vi "KE622x -- Read Trace Buffer.vi"(0 "Resource In":refnum<visa-resource-name>, 1 "Check For SCPI Errors? (T)":bool=TRUE, 7 "Meas Elements To Return":T1={"Timstamp?"=TRUE, "Reading Num?"=TRUE, "Source Value?"=FALSE, "Compliance?"=FALSE, "Average Voltage?"=FALSE}, 11 "error in (no error)":errorcluster) -> (4 "Resource Out (dupl)":refnum<visa-resource-name>, 8 "Trace Buf":T2 {"Average Voltage (V)" format="%.3p"; "Source Val (A)" format="%.3p"; "Timestamp (secs)" format="%.3f"; "Reading" format="%.3p"}, 15 "error out":errorcluster)   [LabVIEW 2019, in "Keithley 622x.lvlib"]
doc: "Used to read the contents of the trace buffer. The user can select which elements should be returned. Note that the data format of the returned results (ASCII, Single Precision, or Double Precision) is automatically detected and handled appropriately so that the user doesn't need to know this information beforehand."
uses:
  Keithley 622x.lvlib
  Configure/Trace Buf/Low Level/Typedefs/KE622x -- Trace Buf.ctl
  Configure/Format/Typedefs/KE622x -- Optional Meas Elements.ctl
  Configure/Trace Buf/Low Level/Typedefs/KE622x -- Trace Buf Readings Type.ctl
panel:
  out "Select Code Dec":u32 format="%0d"
  out "Max Num Bytes To Read":u32
  out "Read String Length":i32
  out "Select Code Bin":u32 format="%06b"
  out "read buffer":string
  # "*** NOTE:  \"Average Voltage\"\nis only available for Differential\nConductance measurements."
  # "*** NOTE:  \"Average Voltage\"\nis only available for Differential\nConductance measurements."
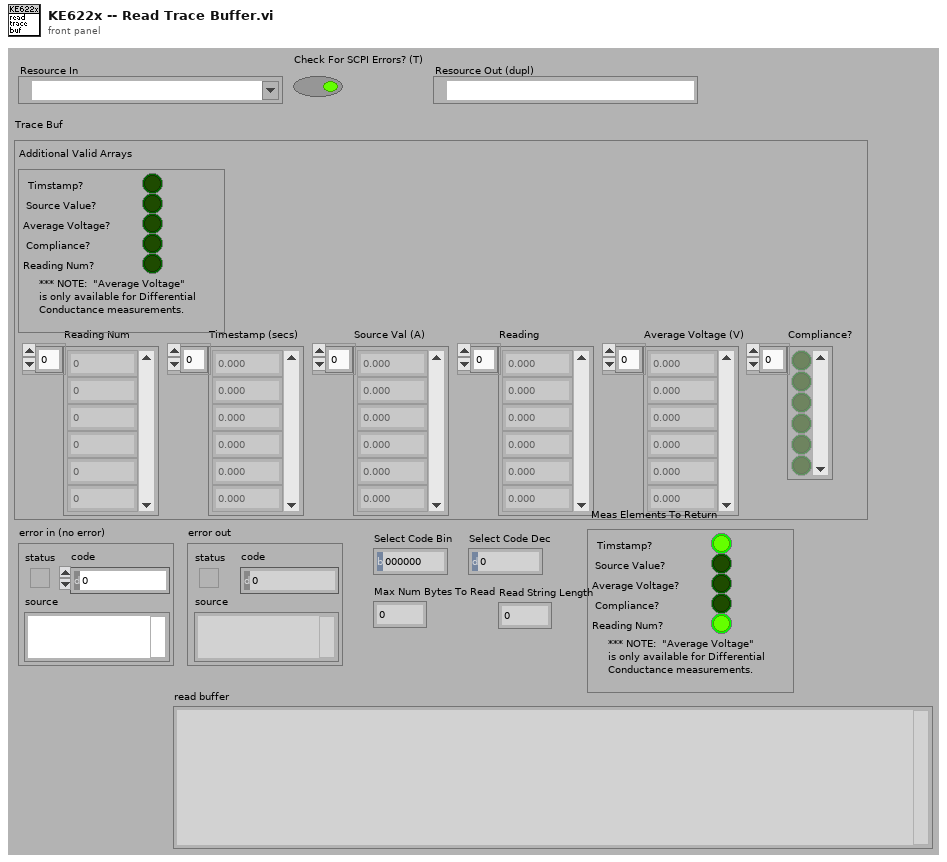
[diagram p1: front panel]
types:
  T1 = typedef "Keithley 622x.lvlib/KE622x -- Optional Meas Elements.ctl" = cluster{"Timstamp?":bool, "Reading Num?":bool, "Source Value?":bool, "Compliance?":bool, "Average Voltage?":bool}
  T2 = typedef "Keithley 622x.lvlib/KE622x -- Trace Buf.ctl" = cluster{"Additional Valid Arrays":T1, "Reading Num":u32[], "Timestamp (secs)":sgl[], "Source Val (A)":sgl[], "Reading":sgl[], "Average Voltage (V)":sgl[], "Compliance?":bool[]}
  T3 = typedef "Keithley 622x.lvlib/KE622x -- Trace Buf Readings Type.ctl" = enum16{"None", "Delta", "Differential Cond", "Pulse Delta"}
  T4 = enum16{"big-endian, network order", "native, host order", "little-endian"}
  T5 = typedef "Keithley 622x.lvlib/KE622x -- Results Format.ctl" = cluster{"Results Format":enum16{"ASCII", "Single Prec Bin", "Double Prec Bin"}, "Bin Byte Order":enum16{"Normal", "Swapped"}}
  T6 = enum16{"ASCII", "Single Prec Bin", "Double Prec Bin"}
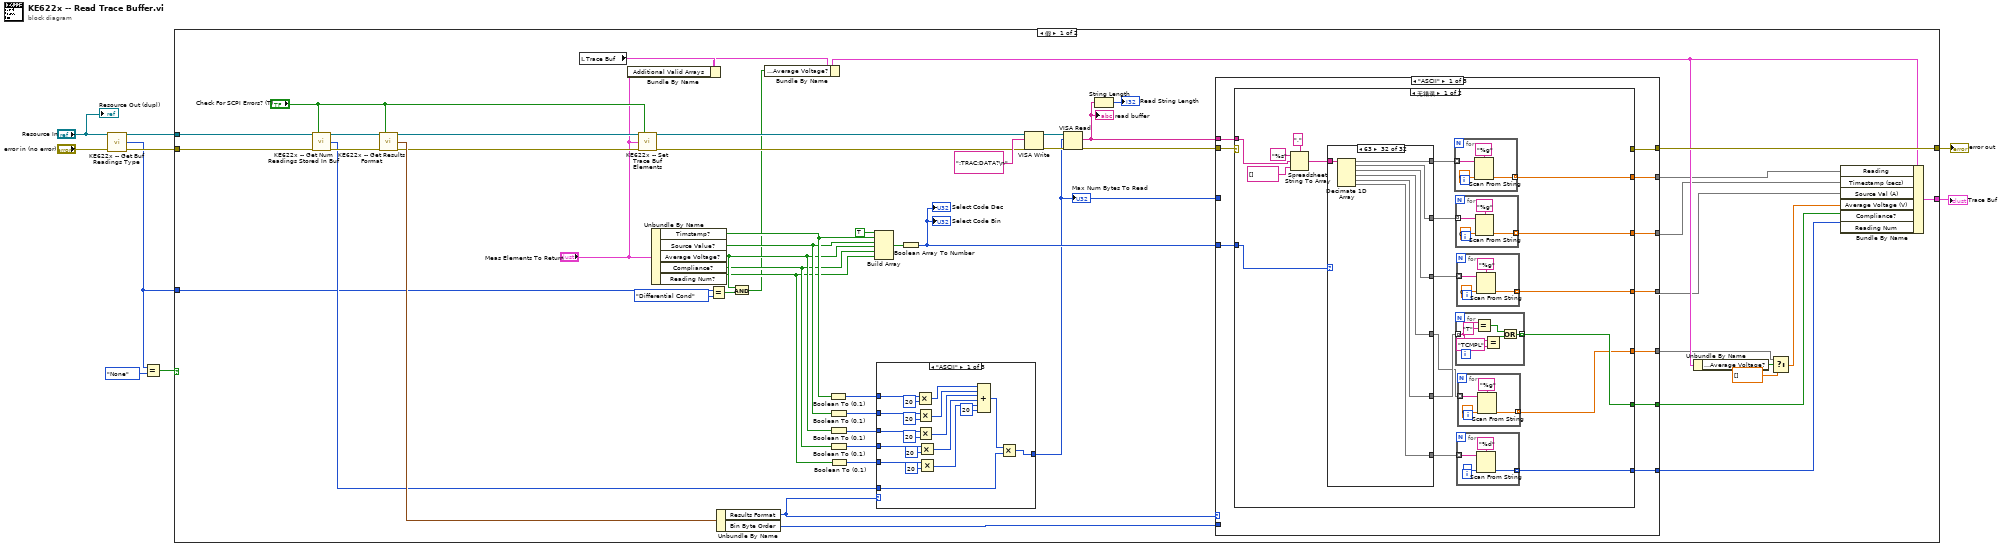
[diagram p0: block diagram]
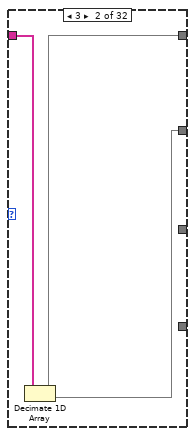
[diagram p3: hidden frame]
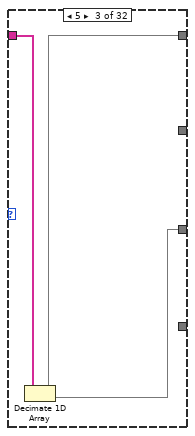
[diagram p4: hidden frame]
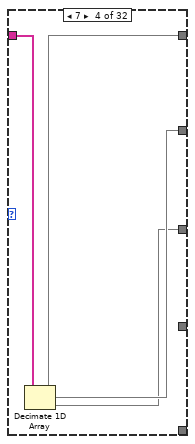
[diagram p5: hidden frame]
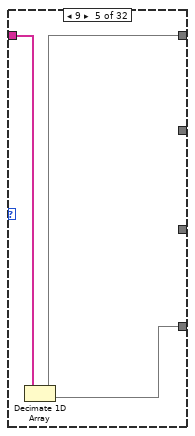
[diagram p6: hidden frame]
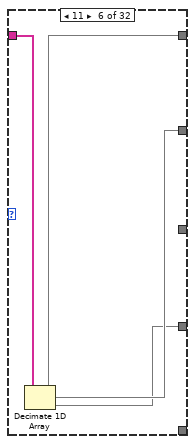
[diagram p7: hidden frame]
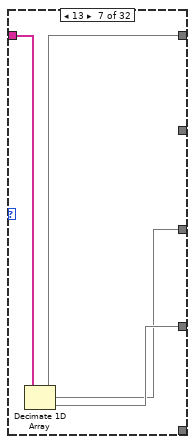
[diagram p8: hidden frame]
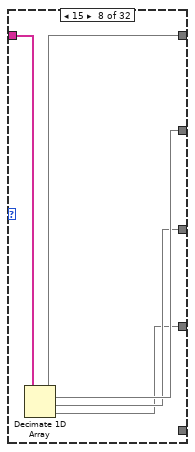
[diagram p9: hidden frame]
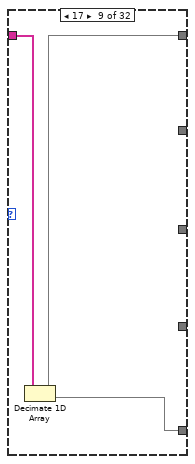
[diagram p10: hidden frame]
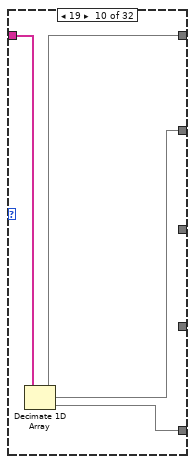
[diagram p11: hidden frame]
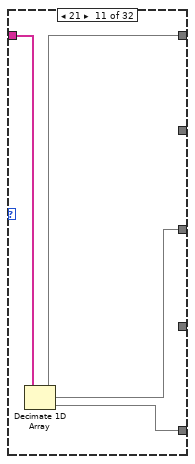
[diagram p12: hidden frame]
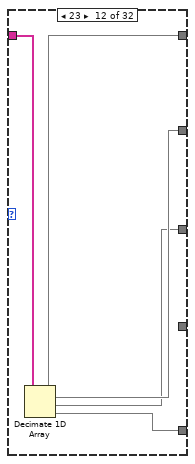
[diagram p13: hidden frame]
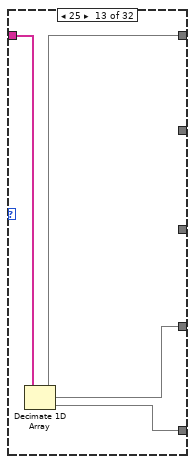
[diagram p14: hidden frame]
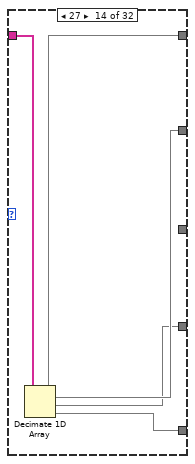
[diagram p15: hidden frame]
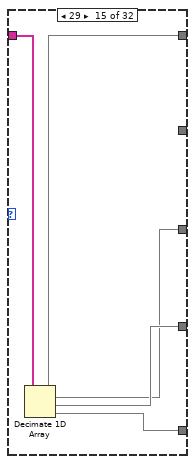
[diagram p16: hidden frame]
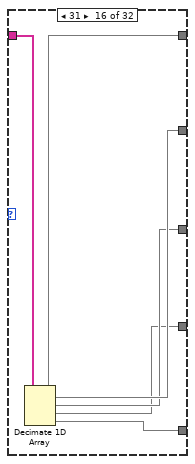
[diagram p17: hidden frame]
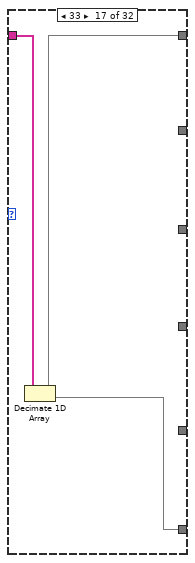
[diagram p18: hidden frame]
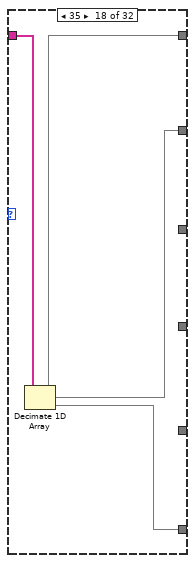
[diagram p19: hidden frame]
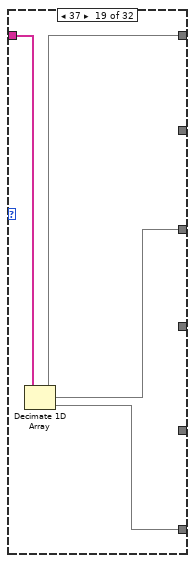
[diagram p20: hidden frame]
diagram:
  n1 = call "KE622x -- Get Buf Readings Type.vi"("Resource In"="Resource In", "error in (no error)"="error in (no error)") -> ("Resource Out (dupl)"=w5:refnum<visa-resource-name>, "Readings Type"=w4:T3, "error out"=w6:errorcluster)  [unwired: 11 in]
  n2 = Equal?(x=w4, y=KE622x_--_Trace_Buf_Readings_Type."None") -> (x = y?=w8:bool)
  n3 = case shown="假" w8 {
    tunnel: w6 -> [w54 w675]
    tunnel: w5 -> [w55 _]
    tunnel: w4 -> [w53 _]
    tunnel: [w25 w673] -> w3
    tunnel: [w10 _] -> w2
    frame False {
      n4 = call "KE622x -- Get Num Readings Stored In Buf.vi"("Resource In"=w55, "Check For SCPI Errors? (T)"="Check For SCPI Errors? (T)", "error in (no error)"=w54) -> ("Resource Out (dupl)"=w60:refnum<visa-resource-name>, "Num Readings Stored"=w57:u32, "error out"=w59:errorcluster)  [unwired: 10 in]
      n5 = call "KE622x -- Get Results Format.vi"("Resource In"=w60, "Check For SCPI Errors? (T)"="Check For SCPI Errors? (T)", "error in (no error)"=w59) -> ("Resource Out (dupl)"=w56:refnum<visa-resource-name>, "Results Format"=w61:T5, "error out"=w58:errorcluster)  [unwired: 10 in]
      n6 = local read "Trace Buf"() -> (w24:T2)
      n7 = Bundle By Name(cluster=w24, "Additional Valid Arrays"="Meas Elements To Return") -> (w21:T2)
      n8 = call "KE622x -- Set Trace Buf Elements.vi"("Resource In"=w56, "Check For SCPI Errors? (T)"="Check For SCPI Errors? (T)", "Meas Elements To Return"="Meas Elements To Return", "error in (no error)"=w58) -> ("Resource Out (dupl)"=w50:refnum<visa-resource-name>, "error out"=w49:errorcluster)  [unwired: 10 in]
      n9 = Unbundle By Name("Meas Elements To Return") -> ("Timstamp?"=w38:bool, "Source Value?"=w37:bool, "Average Voltage?"=w36:bool, "Compliance?"=w35:bool, "Reading Num?"=w34:bool)
      n10 = Equal?(x=w53, y=KE622x_--_Trace_Buf_Readings_Type."Differential Cond") -> (x = y?=w44:bool)
      n11 = Unbundle By Name(w61) -> ("Results Format"=w45:T6, "Bin Byte Order"=w27:enum16{"Normal", "Swapped"})
      n12 = And(x=w36, y=w44) -> (x .and. y?=w22:bool)
      n13 = Bundle By Name(cluster=w21, "Additional Valid Arrays.Average Voltage?"=w22) -> (w20:T2)
      n14 = Boolean To (0,1)(Boolean=w38) -> (0, 1=w43:i16)
      n15 = Boolean To (0,1)(Boolean=w37) -> (0, 1=w42:i16)
      n16 = Boolean To (0,1)(Boolean=w36) -> (0, 1=w41:i16)
      n17 = Boolean To (0,1)(Boolean=w35) -> (0, 1=w40:i16)
      n18 = Boolean To (0,1)(Boolean=w34) -> (0, 1=w39:i16)
      n19 = Build Array(TRUE ("element"), w38, w37, w36, w35, w34) -> (w33:bool[])
      n20 = case shown="\"ASCII\"" w45 {
        tunnel: w57 -> [w615 w636 w657]
        tunnel: w43 -> [w630 w651 w672]
        tunnel: w42 -> [w628 w649 w670]
        tunnel: w41 -> [w625 w646 w667]
        tunnel: w40 -> [w623 w644 w665]
        tunnel: w39 -> [w621 w642 w663]
        tunnel: [w612 w631 w652] -> w28
        frame "ASCII" {
          n21 = Multiply(x=w630, y=i16 20) -> (x*y=w620:i16)
          n22 = Multiply(x=w628, y=i16 20) -> (x*y=w619:i16)
          n23 = Multiply(x=w625, y=i16 20) -> (x*y=w618:i16)
          n24 = Multiply(x=w623, y=i16 20) -> (x*y=w617:i16)
          n25 = Multiply(x=w621, y=i16 20) -> (x*y=w616:i16)
          n26 = Compound Arithmetic op=ADD(w620, w619, w618, w617, w616, i16 20 ("value")) -> (w614:i16)
          n27 = Multiply(x=w614, y=w615) -> (x*y=w612:u32)
        }
        frame "Single Prec Bin" {
          n28 = Multiply(x=w651, y=i16 4) -> (x*y=w641:i16)
          n29 = Multiply(x=w649, y=i16 4) -> (x*y=w640:i16)
          n30 = Multiply(x=w646, y=i16 4) -> (x*y=w639:i16)
          n31 = Multiply(x=w644, y=i16 4) -> (x*y=w638:i16)
          n32 = Multiply(x=w642, y=i16 4) -> (x*y=w637:i16)
          n33 = Compound Arithmetic op=ADD(w641, w640, w639, w638, w637, i16 4 ("value")) -> (w635:i16)
          n34 = Multiply(x=w635, y=w636) -> (x*y=w633:u32)
          n35 = Add(x=w633, y=u32 3) -> (x+y=w631:u32)
        }
        frame "Double Prec Bin" {
          n36 = Multiply(x=w672, y=i16 8) -> (x*y=w662:i16)
          n37 = Multiply(x=w670, y=i16 8) -> (x*y=w661:i16)
          n38 = Multiply(x=w667, y=i16 8) -> (x*y=w660:i16)
          n39 = Multiply(x=w665, y=i16 8) -> (x*y=w659:i16)
          n40 = Multiply(x=w663, y=i16 8) -> (x*y=w658:i16)
          n41 = Compound Arithmetic op=ADD(w662, w661, w660, w659, w658, i16 8 ("value")) -> (w656:i16)
          n42 = Multiply(x=w656, y=w657) -> (x*y=w654:u32)
          n43 = Add(x=w654, y=u32 3) -> (x+y=w652:u32)
        }
      }
      "Max Num Bytes To Read" <- w28
      n44 = Boolean Array To Number(Boolean array=w33) -> (number=w29:u32)
      "Select Code Bin" <- w29
      "Select Code Dec" <- w29
      n45 = VISA Write(VISA resource name=w50, write buffer=":TRAC:DATA?\n", error in (no error)=w49) -> (VISA resource name out=w48:refnum<visa-resource-name>, error out=w47:errorcluster)  [unwired: 1 out]
      n46 = VISA Read(VISA resource name=w48, byte count=w28, error in (no error)=w47) -> (read buffer=w32:string, error out=w26:errorcluster)  [unwired: 2 out]
      "read buffer" <- w32
      n47 = String Length(string=w32) -> (length=→"Read String Length":i32)
      n48 = case shown="\"ASCII\"" w45 {
        tunnel: w32 -> [w71 w269 w443]
        tunnel: w29 -> [w70 w270 w444]
        tunnel: w28 -> [_ _ _]
        tunnel: w27 -> [_ w268 w442]
        tunnel: w26 -> [w69 w267 w441]
        tunnel: [w68 w260 w434] -> w25
        tunnel: [w67 w266 w440] -> w16
        tunnel: [w66 w265 w439] -> w15
        tunnel: [w65 w264 w438] -> w14
        tunnel: [w64 w261 w435] -> w11
        tunnel: [w63 w262 w436] -> w12
        tunnel: [w62 w263 w437] -> w18
        frame "ASCII" {
          n49 = case shown="无错误" w69 {
            selector: w69 -> [_ w259]
            tunnel: w71 -> [w89 _]
            tunnel: w70 -> [w85 _]
            tunnel: [w79 _] -> w67
            tunnel: [w78 _] -> w66
            tunnel: [w77 _] -> w65
            tunnel: [_ w259] -> w68
            tunnel: [w76 _] -> w64
            tunnel: [w75 _] -> w63
            tunnel: [w74 _] -> w62
            frame No Error {
              n50 = Spreadsheet String To Array(delimiter (Tab)=",", format string="%s", spreadsheet string=w89, array type (2D Dbl)=string[] []) -> (array=w84:string[])
              n51 = case shown="63" w85 {
                tunnel: w84 -> [w116 w119 w122 w126 w129 w133 w137 w142 w145 w149 w153 w158 w162 w167 w172 w178 w181 w185 w189 w194 w198 w203 w208 w214 w218 w223 w228 w234 w239 w245 w251 w258]
                tunnel: [w116 w118 w121 w125 w128 w132 w136 w141 w144 w148 w152 w157 w161 w166 w171 w177 w180 w184 w188 w193 w197 w202 w207 w213 w217 w222 w227 w233 w238 w244 w250 w257] -> w83
                tunnel: [_ w117 _ w124 _ w131 _ w140 _ w147 _ w156 _ w165 _ w176 _ w183 _ w192 _ w201 _ w212 _ w219 _ w232 _ w240 _ w256] -> w82
                tunnel: [_ _ w120 w123 _ _ w134 w139 _ _ w150 w155 _ _ w168 w175 _ _ w186 w191 _ _ w204 w211 _ _ w225 w231 _ _ w246 w255] -> w81
                tunnel: [_ _ _ _ w127 w130 w135 w138 _ _ _ _ w160 w164 w170 w174 _ _ _ _ w196 w199 w205 w210 _ _ _ _ w235 w241 w247 w254] -> w72
                tunnel: [_ _ _ _ _ _ _ _ w143 w146 w151 w154 w159 w163 w169 w173 _ _ _ _ _ _ _ _ w215 w220 w224 w230 w236 w242 w248 w253] -> w73
                tunnel: [_ _ _ _ _ _ _ _ _ _ _ _ _ _ _ _ w179 w182 w187 w190 w195 w200 w206 w209 w216 w221 w226 w229 w237 w243 w249 w252] -> w80
                frame 1, Default {
                }
                frame 3 {
                  n52 = Decimate 1D Array(w119) -> (w118:string[], w117:string[])
                }
                frame 5 {
                  n53 = Decimate 1D Array(w122) -> (w121:string[], w120:string[])
                }
                frame 7 {
                  n54 = Decimate 1D Array(w126) -> (w125:string[], w124:string[], w123:string[])
                }
                frame 9 {
                  n55 = Decimate 1D Array(w129) -> (w128:string[], w127:string[])
                }
                frame 11 {
                  n56 = Decimate 1D Array(w133) -> (w132:string[], w131:string[], w130:string[])
                }
                frame 13 {
                  n57 = Decimate 1D Array(w137) -> (w136:string[], w134:string[], w135:string[])
                }
                frame 15 {
                  n58 = Decimate 1D Array(w142) -> (w141:string[], w140:string[], w139:string[], w138:string[])
                }
                frame 17 {
                  n59 = Decimate 1D Array(w145) -> (w144:string[], w143:string[])
                }
                frame 19 {
                  n60 = Decimate 1D Array(w149) -> (w148:string[], w147:string[], w146:string[])
                }
                frame 21 {
                  n61 = Decimate 1D Array(w153) -> (w152:string[], w150:string[], w151:string[])
                }
                frame 23 {
                  n62 = Decimate 1D Array(w158) -> (w157:string[], w156:string[], w155:string[], w154:string[])
                }
                frame 25 {
                  n63 = Decimate 1D Array(w162) -> (w161:string[], w160:string[], w159:string[])
                }
                frame 27 {
                  n64 = Decimate 1D Array(w167) -> (w166:string[], w165:string[], w164:string[], w163:string[])
                }
                frame 29 {
                  n65 = Decimate 1D Array(w172) -> (w171:string[], w168:string[], w170:string[], w169:string[])
                }
                frame 31 {
                  n66 = Decimate 1D Array(w178) -> (w177:string[], w176:string[], w175:string[], w174:string[], w173:string[])
                }
                frame 33 {
                  n67 = Decimate 1D Array(w181) -> (w180:string[], w179:string[])
                }
                frame 35 {
                  n68 = Decimate 1D Array(w185) -> (w184:string[], w183:string[], w182:string[])
                }
                frame 37 {
                  n69 = Decimate 1D Array(w189) -> (w188:string[], w186:string[], w187:string[])
                }
                frame 39 {
                  n70 = Decimate 1D Array(w194) -> (w193:string[], w192:string[], w191:string[], w190:string[])
                }
                frame 41 {
                  n71 = Decimate 1D Array(w198) -> (w197:string[], w196:string[], w195:string[])
                }
                frame 43 {
                  n72 = Decimate 1D Array(w203) -> (w202:string[], w201:string[], w199:string[], w200:string[])
                }
                frame 45 {
                  n73 = Decimate 1D Array(w208) -> (w207:string[], w204:string[], w205:string[], w206:string[])
                }
                frame 47 {
                  n74 = Decimate 1D Array(w214) -> (w213:string[], w212:string[], w211:string[], w210:string[], w209:string[])
                }
                frame 49 {
                  n75 = Decimate 1D Array(w218) -> (w217:string[], w215:string[], w216:string[])
                }
                frame 51 {
                  n76 = Decimate 1D Array(w223) -> (w222:string[], w219:string[], w220:string[], w221:string[])
                }
                frame 53 {
                  n77 = Decimate 1D Array(w228) -> (w227:string[], w225:string[], w224:string[], w226:string[])
                }
                frame 55 {
                  n78 = Decimate 1D Array(w234) -> (w233:string[], w232:string[], w231:string[], w230:string[], w229:string[])
                }
                frame 57 {
                  n79 = Decimate 1D Array(w239) -> (w238:string[], w235:string[], w236:string[], w237:string[])
                }
                frame 59 {
                  n80 = Decimate 1D Array(w245) -> (w244:string[], w240:string[], w241:string[], w242:string[], w243:string[])
                }
                frame 61 {
                  n81 = Decimate 1D Array(w251) -> (w250:string[], w246:string[], w247:string[], w248:string[], w249:string[])
                }
                frame 63 {
                  n82 = Decimate 1D Array(w258) -> (w257:string[], w256:string[], w255:string[], w254:string[], w253:string[], w252:string[])
                }
              }
              n83 = for {
                tunnel: w83 -> [w115] mode=indexing
                tunnel: [w112] -> w79 mode=indexing
                n84 = Scan From String(format string="%g", input string=w115, default 1=sgl 0.0 ("default value 1")) -> (output 1=w112:sgl)  [unwired: 2 in, 3 out]
              }
              n85 = for {
                tunnel: w82 -> [w111] mode=indexing
                tunnel: [w108] -> w78 mode=indexing
                n86 = Scan From String(format string="%g", input string=w111, default 1=sgl 0.0 ("default value 1")) -> (output 1=w108:sgl)  [unwired: 2 in, 3 out]
              }
              n87 = for {
                tunnel: w73 -> [w102] mode=indexing
                tunnel: [w98] -> w75 mode=indexing
                n88 = Equal?(x=w102, y="T") -> (x = y?=w99:bool)
                n89 = Equal?(x=w102, y="TCMPL") -> (x = y?=w100:bool)
                n90 = Or(x=w99, y=w100) -> (x .or. y?=w98:bool)
              }
              n91 = for {
                tunnel: w81 -> [w107] mode=indexing
                tunnel: [w104] -> w77 mode=indexing
                n92 = Scan From String(format string="%g", input string=w107, default 1=sgl 0.0 ("default value 1")) -> (output 1=w104:sgl)  [unwired: 2 in, 3 out]
              }
              n93 = for {
                tunnel: w80 -> [w93] mode=indexing
                tunnel: [w90] -> w76 mode=indexing
                n94 = Scan From String(format string="%d", input string=w93, default 1=u32 0 ("default value 1")) -> (output 1=w90:u32)  [unwired: 2 in, 3 out]
              }
              n95 = for {
                tunnel: w72 -> [w97] mode=indexing
                tunnel: [w94] -> w74 mode=indexing
                n96 = Scan From String(format string="%g", input string=w97, default 1=sgl 0.0 ("default value 1")) -> (output 1=w94:sgl)  [unwired: 2 in, 3 out]
              }
            }
            frame Error {
            }
          }
        }
        frame "Single Prec Bin" {
          n97 = case shown="无错误" w267 {
            selector: w267 -> [_ w433]
            tunnel: w270 -> [w287 _]
            tunnel: w269 -> [w286 _]
            tunnel: w268 -> [w281 _]
            tunnel: [w278 _] -> w266
            tunnel: [w277 _] -> w265
            tunnel: [w276 _] -> w264
            tunnel: [w275 _] -> w263
            tunnel: [w273 _] -> w262
            tunnel: [w271 _] -> w261
            tunnel: [_ w433] -> w260
            frame No Error {
              n98 = case shown="\"Normal\"" w281 {
                tunnel: [T4."big-endian, network order" ("byte order (0:big-endian, network order)") T4."little-endian" ("byte order (0:big-endian, network order)")] -> w280
                frame "Normal" {
                }
                frame "Swapped" {
                }
              }
              n99 = String Subset(string=w286, offset (0)=2) -> (substring=w284:string)  [unwired: 1 in]
              n100 = Unflatten From String(type=sgl[] [], binary string=w284, data includes array or string size? (T)=FALSE, byte order (0:big-endian, network order)=w280) -> (value=w279:sgl[])  [unwired: 1 in, 2 out]
              n101 = case shown="63" w287 {
                tunnel: w279 -> [w290 w293 w296 w300 w303 w307 w311 w316 w319 w323 w327 w332 w336 w341 w346 w352 w355 w359 w363 w368 w372 w377 w382 w388 w392 w397 w402 w408 w413 w419 w425 w432]
                tunnel: [w290 w292 w295 w299 w302 w306 w310 w315 w318 w322 w326 w331 w335 w340 w345 w351 w354 w358 w362 w367 w371 w376 w381 w387 w391 w396 w401 w407 w412 w418 w424 w431] -> w278
                tunnel: [_ w291 _ w298 _ w305 _ w314 _ w321 _ w330 _ w339 _ w350 _ w357 _ w366 _ w375 _ w386 _ w393 _ w406 _ w414 _ w430] -> w277
                tunnel: [_ _ w294 w297 _ _ w308 w313 _ _ w324 w329 _ _ w342 w349 _ _ w360 w365 _ _ w378 w385 _ _ w399 w405 _ _ w420 w429] -> w276
                tunnel: [_ _ _ _ w301 w304 w309 w312 _ _ _ _ w334 w338 w344 w348 _ _ _ _ w370 w373 w379 w384 _ _ _ _ w409 w415 w421 w428] -> w275
                tunnel: [_ _ _ _ _ _ _ _ w317 w320 w325 w328 w333 w337 w343 w347 _ _ _ _ _ _ _ _ w389 w394 w398 w404 w410 w416 w422 w427] -> w274
                tunnel: [_ _ _ _ _ _ _ _ _ _ _ _ _ _ _ _ w353 w356 w361 w364 w369 w374 w380 w383 w390 w395 w400 w403 w411 w417 w423 w426] -> w272
                frame 1, Default {
                }
                frame 3 {
                  n102 = Decimate 1D Array(w293) -> (w292:sgl[], w291:sgl[])
                }
                frame 5 {
                  n103 = Decimate 1D Array(w296) -> (w295:sgl[], w294:sgl[])
                }
                frame 7 {
                  n104 = Decimate 1D Array(w300) -> (w299:sgl[], w298:sgl[], w297:sgl[])
                }
                frame 9 {
                  n105 = Decimate 1D Array(w303) -> (w302:sgl[], w301:sgl[])
                }
                frame 11 {
                  n106 = Decimate 1D Array(w307) -> (w306:sgl[], w305:sgl[], w304:sgl[])
                }
                frame 13 {
                  n107 = Decimate 1D Array(w311) -> (w310:sgl[], w308:sgl[], w309:sgl[])
                }
                frame 15 {
                  n108 = Decimate 1D Array(w316) -> (w315:sgl[], w314:sgl[], w313:sgl[], w312:sgl[])
                }
                frame 17 {
                  n109 = Decimate 1D Array(w319) -> (w318:sgl[], w317:sgl[])
                }
                frame 19 {
                  n110 = Decimate 1D Array(w323) -> (w322:sgl[], w321:sgl[], w320:sgl[])
                }
                frame 21 {
                  n111 = Decimate 1D Array(w327) -> (w326:sgl[], w324:sgl[], w325:sgl[])
                }
                frame 23 {
                  n112 = Decimate 1D Array(w332) -> (w331:sgl[], w330:sgl[], w329:sgl[], w328:sgl[])
                }
                frame 25 {
                  n113 = Decimate 1D Array(w336) -> (w335:sgl[], w334:sgl[], w333:sgl[])
                }
                frame 27 {
                  n114 = Decimate 1D Array(w341) -> (w340:sgl[], w339:sgl[], w338:sgl[], w337:sgl[])
                }
                frame 29 {
                  n115 = Decimate 1D Array(w346) -> (w345:sgl[], w342:sgl[], w344:sgl[], w343:sgl[])
                }
                frame 31 {
                  n116 = Decimate 1D Array(w352) -> (w351:sgl[], w350:sgl[], w349:sgl[], w348:sgl[], w347:sgl[])
                }
                frame 33 {
                  n117 = Decimate 1D Array(w355) -> (w354:sgl[], w353:sgl[])
                }
                frame 35 {
                  n118 = Decimate 1D Array(w359) -> (w358:sgl[], w357:sgl[], w356:sgl[])
                }
                frame 37 {
                  n119 = Decimate 1D Array(w363) -> (w362:sgl[], w360:sgl[], w361:sgl[])
                }
                frame 39 {
                  n120 = Decimate 1D Array(w368) -> (w367:sgl[], w366:sgl[], w365:sgl[], w364:sgl[])
                }
                frame 41 {
                  n121 = Decimate 1D Array(w372) -> (w371:sgl[], w370:sgl[], w369:sgl[])
                }
                frame 43 {
                  n122 = Decimate 1D Array(w377) -> (w376:sgl[], w375:sgl[], w373:sgl[], w374:sgl[])
                }
                frame 45 {
                  n123 = Decimate 1D Array(w382) -> (w381:sgl[], w378:sgl[], w379:sgl[], w380:sgl[])
                }
                frame 47 {
                  n124 = Decimate 1D Array(w388) -> (w387:sgl[], w386:sgl[], w385:sgl[], w384:sgl[], w383:sgl[])
                }
                frame 49 {
                  n125 = Decimate 1D Array(w392) -> (w391:sgl[], w389:sgl[], w390:sgl[])
                }
                frame 51 {
                  n126 = Decimate 1D Array(w397) -> (w396:sgl[], w393:sgl[], w394:sgl[], w395:sgl[])
                }
                frame 53 {
                  n127 = Decimate 1D Array(w402) -> (w401:sgl[], w399:sgl[], w398:sgl[], w400:sgl[])
                }
                frame 55 {
                  n128 = Decimate 1D Array(w408) -> (w407:sgl[], w406:sgl[], w405:sgl[], w404:sgl[], w403:sgl[])
                }
                frame 57 {
                  n129 = Decimate 1D Array(w413) -> (w412:sgl[], w409:sgl[], w410:sgl[], w411:sgl[])
                }
                frame 59 {
                  n130 = Decimate 1D Array(w419) -> (w418:sgl[], w414:sgl[], w415:sgl[], w416:sgl[], w417:sgl[])
                }
                frame 61 {
                  n131 = Decimate 1D Array(w425) -> (w424:sgl[], w420:sgl[], w421:sgl[], w422:sgl[], w423:sgl[])
                }
                frame 63 {
                  n132 = Decimate 1D Array(w432) -> (w431:sgl[], w430:sgl[], w429:sgl[], w428:sgl[], w427:sgl[], w426:sgl[])
                }
              }
              n133 = Not Equal To 0?(x=w274) -> (x != 0?=w273:bool[])
              n134 = To Unsigned Long Integer(number=w272) -> (unsigned 32bit integer=w271:u32[])
            }
            frame Error {
            }
          }
        }
        frame "Double Prec Bin" {
          n135 = case shown="无错误" w441 {
            selector: w441 -> [_ w611]
            tunnel: w444 -> [w465 _]
            tunnel: w443 -> [w464 _]
            tunnel: w442 -> [w459 _]
            tunnel: [w448 _] -> w440
            tunnel: [w447 _] -> w439
            tunnel: [w446 _] -> w438
            tunnel: [w445 _] -> w437
            tunnel: [w451 _] -> w436
            tunnel: [w449 _] -> w435
            tunnel: [_ w611] -> w434
            frame No Error {
              n136 = case shown="\"Normal\"" w459 {
                tunnel: [T4."big-endian, network order" ("byte order (0:big-endian, network order)") T4."little-endian" ("byte order (0:big-endian, network order)")] -> w458
                frame "Normal" {
                }
                frame "Swapped" {
                }
              }
              n137 = String Subset(string=w464, offset (0)=2) -> (substring=w462:string)  [unwired: 1 in]
              n138 = Unflatten From String(type=dbl[] [], binary string=w462, data includes array or string size? (T)=FALSE, byte order (0:big-endian, network order)=w458) -> (value=w457:dbl[])  [unwired: 1 in, 2 out]
              n139 = case shown="63" w465 {
                tunnel: w457 -> [w468 w471 w474 w478 w481 w485 w489 w494 w497 w501 w505 w510 w514 w519 w524 w530 w533 w537 w541 w546 w550 w555 w560 w566 w570 w575 w580 w586 w591 w597 w603 w610]
                tunnel: [w468 w470 w473 w477 w480 w484 w488 w493 w496 w500 w504 w509 w513 w518 w523 w529 w532 w536 w540 w545 w549 w554 w559 w565 w569 w574 w579 w585 w590 w596 w602 w609] -> w456
                tunnel: [_ w469 _ w476 _ w483 _ w492 _ w499 _ w508 _ w517 _ w528 _ w535 _ w544 _ w553 _ w564 _ w571 _ w584 _ w592 _ w608] -> w455
                tunnel: [_ _ w472 w475 _ _ w486 w491 _ _ w502 w507 _ _ w520 w527 _ _ w538 w543 _ _ w556 w563 _ _ w577 w583 _ _ w598 w607] -> w454
                tunnel: [_ _ _ _ w479 w482 w487 w490 _ _ _ _ w512 w516 w522 w526 _ _ _ _ w548 w551 w557 w562 _ _ _ _ w587 w593 w599 w606] -> w453
                tunnel: [_ _ _ _ _ _ _ _ w495 w498 w503 w506 w511 w515 w521 w525 _ _ _ _ _ _ _ _ w567 w572 w576 w582 w588 w594 w600 w605] -> w452
                tunnel: [_ _ _ _ _ _ _ _ _ _ _ _ _ _ _ _ w531 w534 w539 w542 w547 w552 w558 w561 w568 w573 w578 w581 w589 w595 w601 w604] -> w450
                frame 1, Default {
                }
                frame 3 {
                  n140 = Decimate 1D Array(w471) -> (w470:dbl[], w469:dbl[])
                }
                frame 5 {
                  n141 = Decimate 1D Array(w474) -> (w473:dbl[], w472:dbl[])
                }
                frame 7 {
                  n142 = Decimate 1D Array(w478) -> (w477:dbl[], w476:dbl[], w475:dbl[])
                }
                frame 9 {
                  n143 = Decimate 1D Array(w481) -> (w480:dbl[], w479:dbl[])
                }
                frame 11 {
                  n144 = Decimate 1D Array(w485) -> (w484:dbl[], w483:dbl[], w482:dbl[])
                }
                frame 13 {
                  n145 = Decimate 1D Array(w489) -> (w488:dbl[], w486:dbl[], w487:dbl[])
                }
                frame 15 {
                  n146 = Decimate 1D Array(w494) -> (w493:dbl[], w492:dbl[], w491:dbl[], w490:dbl[])
                }
                frame 17 {
                  n147 = Decimate 1D Array(w497) -> (w496:dbl[], w495:dbl[])
                }
                frame 19 {
                  n148 = Decimate 1D Array(w501) -> (w500:dbl[], w499:dbl[], w498:dbl[])
                }
                frame 21 {
                  n149 = Decimate 1D Array(w505) -> (w504:dbl[], w502:dbl[], w503:dbl[])
                }
                frame 23 {
                  n150 = Decimate 1D Array(w510) -> (w509:dbl[], w508:dbl[], w507:dbl[], w506:dbl[])
                }
                frame 25 {
                  n151 = Decimate 1D Array(w514) -> (w513:dbl[], w512:dbl[], w511:dbl[])
                }
                frame 27 {
                  n152 = Decimate 1D Array(w519) -> (w518:dbl[], w517:dbl[], w516:dbl[], w515:dbl[])
                }
                frame 29 {
                  n153 = Decimate 1D Array(w524) -> (w523:dbl[], w520:dbl[], w522:dbl[], w521:dbl[])
                }
                frame 31 {
                  n154 = Decimate 1D Array(w530) -> (w529:dbl[], w528:dbl[], w527:dbl[], w526:dbl[], w525:dbl[])
                }
                frame 33 {
                  n155 = Decimate 1D Array(w533) -> (w532:dbl[], w531:dbl[])
                }
                frame 35 {
                  n156 = Decimate 1D Array(w537) -> (w536:dbl[], w535:dbl[], w534:dbl[])
                }
                frame 37 {
                  n157 = Decimate 1D Array(w541) -> (w540:dbl[], w538:dbl[], w539:dbl[])
                }
                frame 39 {
                  n158 = Decimate 1D Array(w546) -> (w545:dbl[], w544:dbl[], w543:dbl[], w542:dbl[])
                }
                frame 41 {
                  n159 = Decimate 1D Array(w550) -> (w549:dbl[], w548:dbl[], w547:dbl[])
                }
                frame 43 {
                  n160 = Decimate 1D Array(w555) -> (w554:dbl[], w553:dbl[], w551:dbl[], w552:dbl[])
                }
                frame 45 {
                  n161 = Decimate 1D Array(w560) -> (w559:dbl[], w556:dbl[], w557:dbl[], w558:dbl[])
                }
                frame 47 {
                  n162 = Decimate 1D Array(w566) -> (w565:dbl[], w564:dbl[], w563:dbl[], w562:dbl[], w561:dbl[])
                }
                frame 49 {
                  n163 = Decimate 1D Array(w570) -> (w569:dbl[], w567:dbl[], w568:dbl[])
                }
                frame 51 {
                  n164 = Decimate 1D Array(w575) -> (w574:dbl[], w571:dbl[], w572:dbl[], w573:dbl[])
                }
                frame 53 {
                  n165 = Decimate 1D Array(w580) -> (w579:dbl[], w577:dbl[], w576:dbl[], w578:dbl[])
                }
                frame 55 {
                  n166 = Decimate 1D Array(w586) -> (w585:dbl[], w584:dbl[], w583:dbl[], w582:dbl[], w581:dbl[])
                }
                frame 57 {
                  n167 = Decimate 1D Array(w591) -> (w590:dbl[], w587:dbl[], w588:dbl[], w589:dbl[])
                }
                frame 59 {
                  n168 = Decimate 1D Array(w597) -> (w596:dbl[], w592:dbl[], w593:dbl[], w594:dbl[], w595:dbl[])
                }
                frame 61 {
                  n169 = Decimate 1D Array(w603) -> (w602:dbl[], w598:dbl[], w599:dbl[], w600:dbl[], w601:dbl[])
                }
                frame 63 {
                  n170 = Decimate 1D Array(w610) -> (w609:dbl[], w608:dbl[], w607:dbl[], w606:dbl[], w605:dbl[], w604:dbl[])
                }
              }
              n171 = Not Equal To 0?(x=w452) -> (x != 0?=w451:bool[])
              n172 = To Unsigned Long Integer(number=w450) -> (unsigned 32bit integer=w449:u32[])
              n173 = To Single Precision Float(number=w456) -> (single precision float=w448:sgl[])
              n174 = To Single Precision Float(number=w455) -> (single precision float=w447:sgl[])
              n175 = To Single Precision Float(number=w454) -> (single precision float=w446:sgl[])
              n176 = To Single Precision Float(number=w453) -> (single precision float=w445:sgl[])
            }
            frame Error {
            }
          }
        }
      }
      n177 = Unbundle By Name(w20) -> ("Additional Valid Arrays.Average Voltage?"=w19:bool)
      n178 = Select(t=w18, s=w19, f=sgl[] []) -> (s? t:f=w13:sgl[])
      n179 = Bundle By Name(cluster=w20, "Reading"=w16, "Timestamp (secs)"=w15, "Source Val (A)"=w14, "Average Voltage (V)"=w13, "Compliance?"=w12, "Reading Num"=w11) -> (w10:T2)
    }
    frame True {
      n180 = call <vilib>:"Error Cluster From Error Code.vi"("show call chain? (False)"=TRUE, "error in (no error)"=w675, "error message (\"\")"="Buffer data type is 'NONE', thus\nthere is no data in buffer.", "error code (0)"=-1) -> ("error out"=w673:errorcluster)  [unwired: 5 in]
    }
  }
  "error out" <- w3
  "Trace Buf" <- w2
  "Resource Out (dupl)" <- "Resource In"
